vi "average1.vi"(6 "Size":i32=100, 7 "Signal":waveform(dbl)(graph) caption="Signals") -> (3 "Mean":waveform(i16)(graph))   [LabVIEW 2010]
doc: "Acquires a large number of data points and compresses the data points into a smaller number of points.\n--------------------\n\nThis Express VI is configured as follows:\n\nReduction Factor: 100\nReduction Method: Mean"
panel:
  out "LastIndex":i32
  # "Усреднение с сохранением фазы"
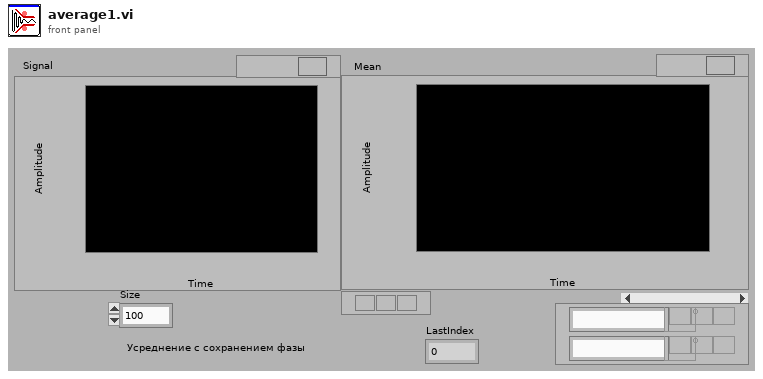
[diagram p1: front panel]
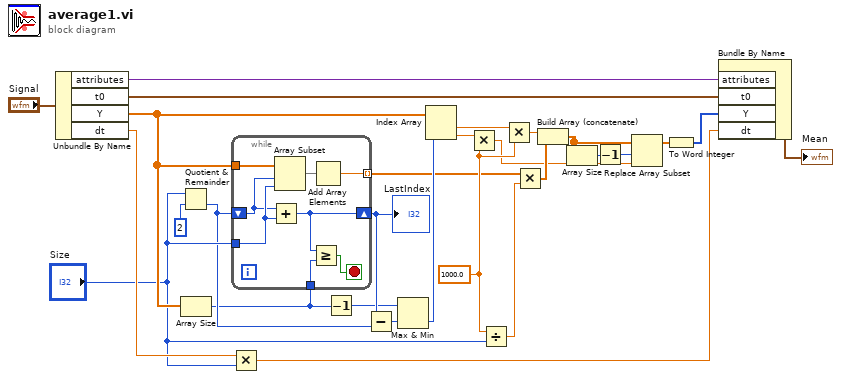
[diagram p0: block diagram]
diagram:
  w12 = 1000.0 ("x")
  n1 = Unbundle By Name("Signal") -> ("attributes"=w3:variant, "t0"=w4:timestamp, "Y"=w27:dbl[], "dt"=w26:dbl)
  n2 = Quotient & Remainder(x="Size", y=2) -> (floor(x/y)=w18:i32)  [unwired: 1 out]
  n3 = Array Size(array=w27) -> (size(s)=w16:i32)
  n4 = Multiply(x=w26, y="Size") -> (x*y=w25:dbl)
  n5 = while {
    tunnel: w27 -> [w35]
    tunnel: [w36] -> w11 mode=indexing
    tunnel: "Size" -> [w33]
    shift-right: [w31] -> w19
    shift-left: w18 -> [w32]
    tunnel: w16 -> [w30]
    stop <- w29 stop-if-true
    n6 = Add(x=w32, y=w33) -> (x+y=w31:i32)
    n7 = Array Subset(array=w35, index=w32, length=w33) -> (w34:dbl[])
    n8 = Greater Or Equal?(x=w31, y=w30) -> (x >= y?=w29:bool)
    n9 = Add Array Elements(numeric array=w34) -> (sum=w36:dbl)
  }
  "LastIndex" <- w19
  n10 = Decrement(x=w16) -> (x-1=w15:i32)
  n11 = Subtract(x=w19, y=w18) -> (x-y=w17:i32)
  n12 = Max & Min(x=w15, y=w17) -> (min(x,y)=w14:i32)  [unwired: 1 out]
  n13 = Index Array(array=w27, index #2=w14) -> (element #1=w22:dbl, element #2=w13:dbl)  [unwired: 1 in]
  n14 = Multiply(x=w13, y=w12) -> (x*y=w7:dbl)
  n15 = Divide(x=w12, y="Size") -> (x/y=w23:dbl)
  n16 = Multiply(x=w22, y=w12) -> (x*y=w21:dbl)
  n17 = Multiply(x=w11, y=w23) -> (x*y=w20:dbl[])
  n18 = Build Array (concatenate)(w21, w20) -> (w10:dbl[])
  n19 = Array Size(array=w10) -> (size(s)=w9:i32)
  n20 = Decrement(x=w9) -> (x-1=w8:i32)
  n21 = Replace Array Subset(array=w10, new element=w7, index=w8) -> (w6:dbl[])
  n22 = To Word Integer(number=w6) -> (16bit integer=w5:i16[])
  n23 = Bundle By Name("attributes"=w3, "t0"=w4, "Y"=w5, "dt"=w25) -> (→"Mean":waveform(i16))  [unwired: 1 in]
